vi "GetCoreChannelProperties.vi"(11 "Channel":T1) -> (3 "Tdms Properties":T4[](array[typedef]))   [LabVIEW 2017, in "Tdms.lvlib"]
uses:
  <vilib>/addons/InsightCM/Utilities/Tdms/Tdms.lvlib
  <vilib>/addons/InsightCM/Utilities/Tdms/controls/Property.ctl
  <vilib>/addons/InsightCM/MessageBus/Base/controls/R2_Channel.ctl
  <vilib>/addons/InsightCM/MessageBus/Base/controls/KeyValuePair.ctl
  <vilib>/addons/InsightCM/MessageBus/Base/controls/Metric.ctl
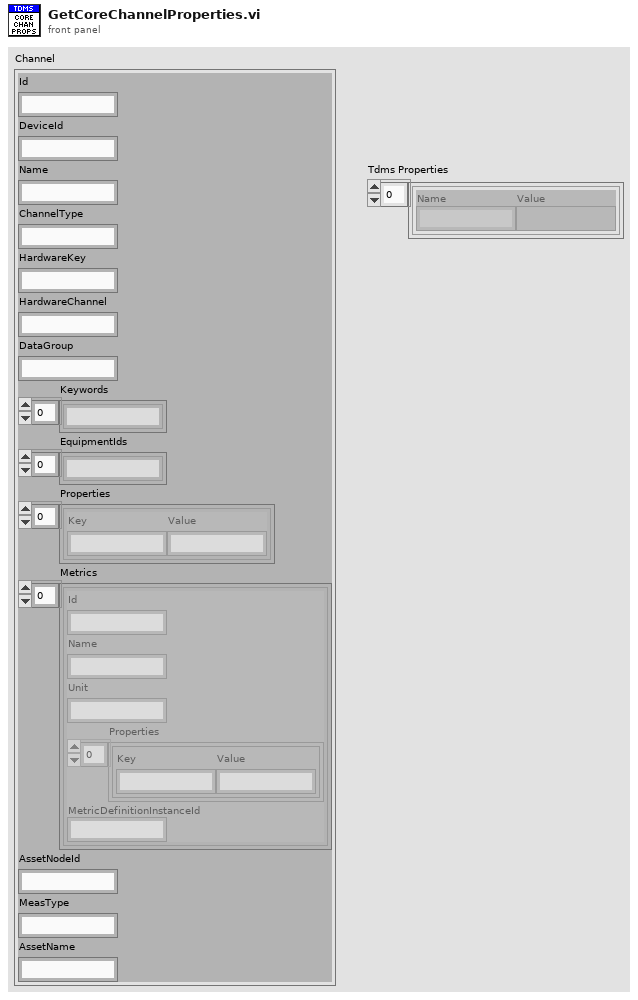
[diagram p1: front panel]
types:
  T1 = typedef "R2_Channel.ctl" = cluster{"Id":string, "DeviceId":string, "Name":string, "ChannelType":string, "HardwareKey":string, "HardwareChannel":string, "DataGroup":string, "Keywords":string[], "EquipmentIds":string[], "Properties":T2[], "Metrics":T3[], "AssetNodeId":string, "MeasType":string, "AssetName":string}
  T2 = typedef "KeyValuePair.ctl" = cluster{"Key":string, "Value":string}
  T3 = typedef "Metric.ctl" = cluster{"Id":string, "Name":string, "Unit":string, "Properties":T2[], "MetricDefinitionInstanceId":string}
  T4 = typedef "Tdms.lvlib/Property.ctl" = cluster{"Name":string, "Value":variant}
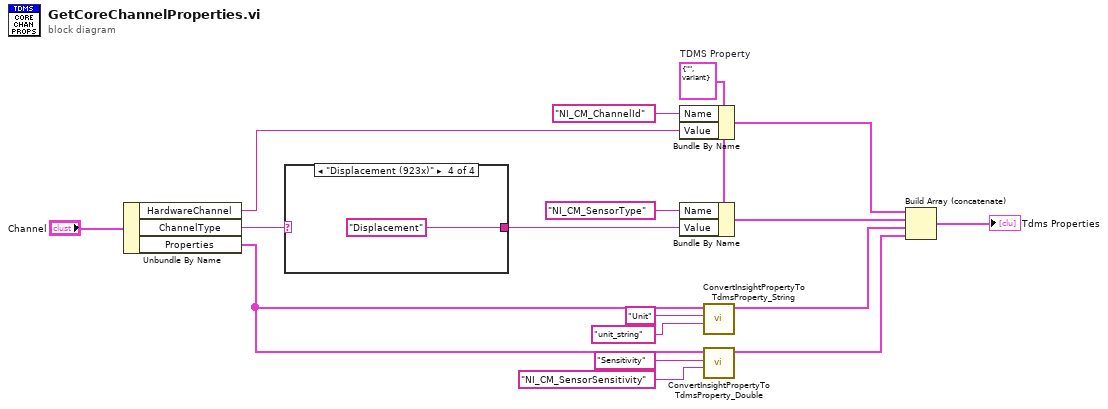
[diagram p0: block diagram]
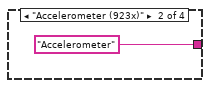
[diagram p3: hidden frame]
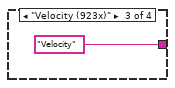
[diagram p4: hidden frame]
diagram:
  w5 = T4 {"Name"="", "Value"=variant}  # TDMS Property
  n1 = Unbundle By Name("Channel") -> ("HardwareChannel"=w7:string, "ChannelType"=w4:string, "Properties"=w6:T2[])
  n2 = case shown="\"Displacement (923x)\"" w4 {
    selector: w4 -> [w18 _ _ _]
    tunnel: [w18 "Accelerometer" ("Name") "Velocity" ("Name") "Displacement" ("Name")] -> w3
    frame Default {
    }
    frame "Accelerometer (923x)" {
    }
    frame "Velocity (923x)" {
    }
    frame "Displacement (923x)" {
    }
  }
  n3 = Bundle By Name(cluster=w5, "Name"="NI_CM_ChannelId", "Value"=w7) -> (w13:T4)
  n4 = Bundle By Name(cluster=w5, "Name"="NI_CM_SensorType", "Value"=w3) -> (w12:T4)
  n5 = call <vilib>:"ConvertInsightPropertyToTdmsProperty_String.vi"("Tdms Property Name"="unit_string", "Insight Property Name"="Unit", "Insight Properties"=w6) -> ("Tdms Properties"=w11:T4[])  [unwired: 8 in]
  n6 = call <vilib>:"ConvertInsightPropertyToTdmsProperty_Double.vi"("Tdms Property Name"="NI_CM_SensorSensitivity" ("Name"), "Insight Property Name"="Sensitivity" ("Name"), "Insight Properties"=w6) -> ("Tdms Properties"=w10:T4[])  [unwired: 8 in]
  n7 = Build Array (concatenate)(w13, w12, w11, w10) -> (→"Tdms Properties":T4[])
